vi "Scan Temp str (SubVI).vi"(6 "字符串":string, 9 "queue out":refnum<queue>, 11 "队列输入":refnum<queue>) -> (0 "错误输出":errorcluster)   [LabVIEW 2019, in "Take Seq.lvlib"]
uses:
  Take Seq.lvlib
  config.ctl
  Instrument.ctl
  lib/QDInstrument.dll
  SubVI.lvlib
panel:
  # "(真是通道1，假是通道2)"
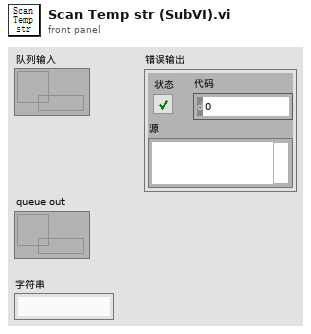
[diagram p1: front panel]
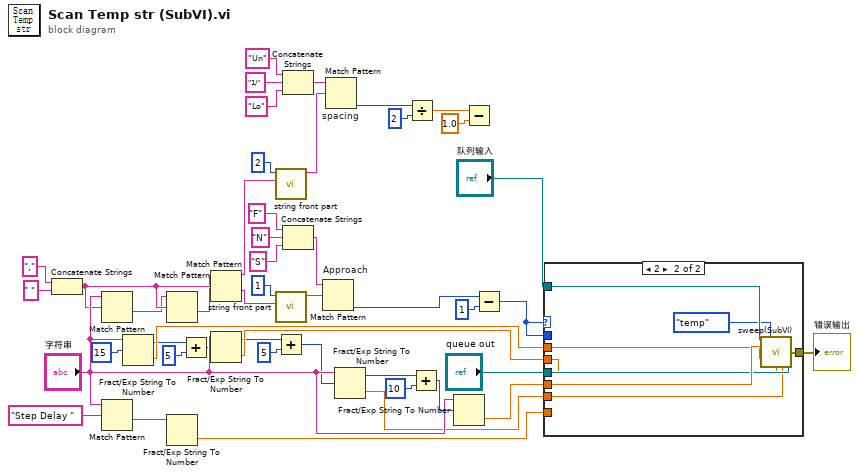
[diagram p0: block diagram]
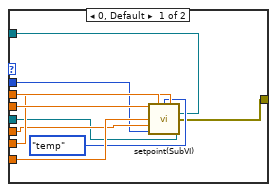
[diagram p2: hidden frame]
diagram:
  n1 = Concatenate Strings("," ("字符串"), " " ("字符串")) -> (w21:string)
  n2 = Match Pattern(string="字符串", regular expression=w21) -> (after substring=w1:string)  [unwired: 1 in, 3 out]
  n3 = Match Pattern(string="字符串", regular expression="Step Delay ") -> (after substring=w44:string)  [unwired: 1 in, 3 out]
  n4 = Fract/Exp String To Number(string="字符串", offset=15 ("偏移量")) -> (offset past number=w3:i32, number=w38:dbl)  [unwired: 2 in]
  n5 = Match Pattern(string=w1, regular expression=w21) -> (after substring=w20:string)  [unwired: 1 in, 3 out]
  n6 = Fract/Exp String To Number(string=w44) -> (number=w45:dbl)  [unwired: 3 in, 1 out]
  n7 = Add(x=w3, y=5) -> (x+y=w4:i32)
  n8 = Match Pattern(string=w20, regular expression=w21) -> (before substring=w22:string, after substring=w34:string)  [unwired: 1 in, 2 out]
  n9 = Fract/Exp String To Number(string="字符串", offset=w4) -> (offset past number=w15:i32, number=w39:dbl)  [unwired: 2 in]
  n10 = call "string front part.vi"("字符串"=w22, "偏移量(0)"=2) -> ("result string"=w24:string)  [unwired: 9 in]
  n11 = call "string front part.vi"("字符串"=w34, "偏移量(0)"=1) -> ("result string"=w7:string)  [unwired: 9 in]
  n12 = Add(x=w15, y=5) -> (x+y=w17:i32)
  n13 = Concatenate Strings("Un" ("字符串"), "1/" ("字符串"), "Lo" ("字符串")) -> (w28:string)
  n14 = Concatenate Strings("F" ("字符串"), "N" ("字符串"), "S" ("字符串")) -> (w10:string)
  n15 = Match Pattern "Approach"(string=w10, regular expression=w7) -> (offset past match=w11:i32)  [unwired: 1 in, 3 out]
  n16 = Match Pattern "spacing"(string=w28, regular expression=w24) -> (offset past match=w29:i32)  [unwired: 1 in, 3 out]
  n17 = Fract/Exp String To Number(string="字符串", offset=w17) -> (offset past number=w33:i32, number=w41:dbl)  [unwired: 2 in]
  n18 = Divide(x=w29, y=2) -> (x/y=w31:dbl)
  n19 = Add(x=w33, y=10) -> (x+y=w19:i32)
  n20 = Fract/Exp String To Number(string="字符串", offset=w19) -> (number=w37:dbl)  [unwired: 2 in, 1 out]
  n21 = Subtract(x=w31, y=1.0) -> ()  [unwired: 1 out]
  n22 = Subtract(x=w11, y=1) -> (x-y=w36:i32)
  n23 = case shown="2" w36 {
    tunnel: w36 -> [w52 _]
    tunnel: w37 -> [w53 w64]
    tunnel: w41 -> [w55 w59]
    tunnel: w38 -> [w56 w63]
    tunnel: w39 -> [w57 w60]
    tunnel: "队列输入" -> [w50 w65]
    tunnel: "queue out" -> [w49 w62]
    tunnel: [w48 w58] -> w43
    tunnel: w45 -> [w54 _]
    frame 0, Default {
      n24 = call "setpoint(SubVI).vi"("Filed 2"=w57, "Field"=w56, "类型"=enum16{"temp", "field", "position"}."temp", "Rate/speed"=w55, "data"=w50, "Delay"=w54, "steps number"=w53, "Approach"=w52, "config"=w49) -> ("错误输出"=w48:errorcluster)  [unwired: 6 in]
    }
    frame 2 {
      n25 = call "sweep(SubVI).vi"("data"=w65, "类型"=enum16{"temp", "field", "position"}."temp", "config"=w62, "steps number"=w64, "Field"=w63, "Field 2"=w60, "Rate、speed"=w59) -> ("错误输出"=w58:errorcluster)  [unwired: 8 in]
    }
  }
  "错误输出" <- w43
